vi "Read Config.vi"(8 "error in (no error)":errorcluster, 11 "AcquistionObject in":refnum<class "AcquistionObject.lvclass">) -> (0 "error out":errorcluster, 2 "config data":T1, 3 "AcquistionObject out":refnum<class "AcquistionObject.lvclass">)   [LabVIEW 2010, in "AcquistionObject.lvclass"]
uses:
  AcquistionObject.lvclass
  <vilib>/Utility/config.llb/Config Data RefNum.ctl
  AcquistionObject.lvclass/AcquistionObject.ctl
  <vilib>/Utility/config.llb/NI_LVConfig.lvlib
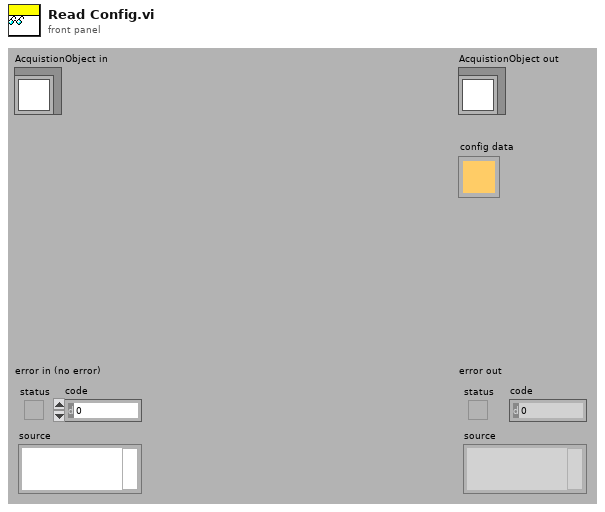
[diagram p1: front panel]
types:
  T1 = typedef "NI_LVConfig.lvlib/Config Data RefNum.ctl" = refnum<k1>
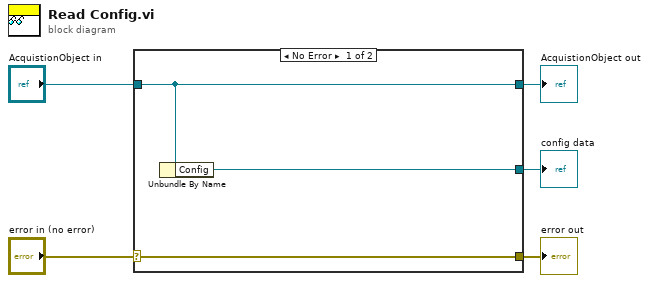
[diagram p0: block diagram]
diagram:
  n1 = case shown="No Error" "error in (no error)" {
    selector: "error in (no error)" -> [w8 w9]
    tunnel: [w8 w9] -> w4
    tunnel: [w7 w10] -> w2
    tunnel: "AcquistionObject in" -> [w7 w10]
    tunnel: [w6 _] -> w1
    frame No Error {
      n2 = Unbundle By Name(w7) -> ("Config"=w6:T1)
    }
    frame Error {
    }
  }
  "error out" <- w4
  "AcquistionObject out" <- w2
  "config data" <- w1
